vi "Configure Target - Legacy.vi"() -> ()   [LabVIEW 2020, in "LMH-LINX.lvlib"]
uses:
  LMH-LINX.lvlib
  Toolbox/LMH-Toolbox.lvlib
  Install LV Events.ctl
  Target Management/Install LV Data.ctl
  Target Management/Target Info.ctl
  Target Management/Status FGV States.ctl
  c:/p4/penguin/lvaddon/MakerHub/LINX/trunk/20.1/objects/MakerHub_LINX/win32U/i386/msvc90/release/LabVIEW/vi.lib/MakerHub/LINX/Resources/Renci.SshNet.dll
  Resources/Renci.SshNet.dll
  Target Management/NIC Info.ctl
  Target Management/NIC Mode.ctl
panel:
  in  "Done":bool
  out "Hostname":string
  out "Status":string
  in  "Hostname":string="raspberrypi"
  in  "Update Hostname":bool
  in  "Password":string="raspberry"
  in  "Username":string="pi"
  in  "Hostname or IP":string="raspberrypi"
  in  "Connect":bool
  out "Event Handler Iterations":i32
  out "Detailed Log":string
  out "Status Log":string
  out "Error Out":errorcluster
  # "Use this wizard to configure target settings for BeagleBone Black and Raspberry Pi 2 devices.\n\n1. Ensure the target is powered on and accessible on the same network as this computer.\n2. Enter the target's current hostname or IP address.\n3. Enter the new target hostname and click Update."
  # "Target Connection Settings"
  # "New Settings"
  # "LINX\nConfigure Target"
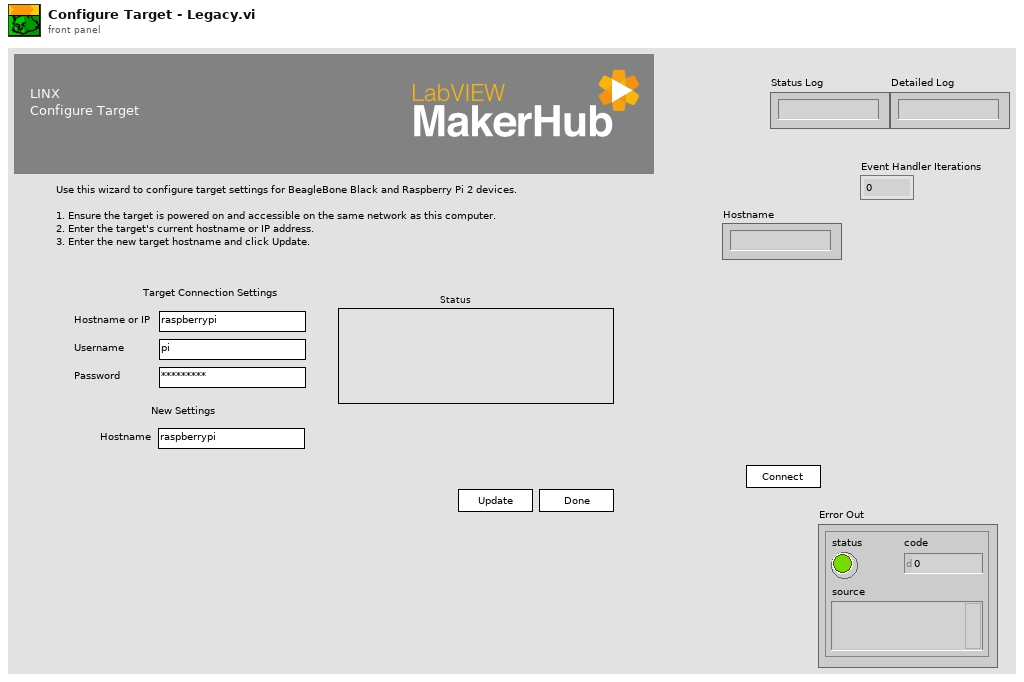
[diagram p1: front panel]
types:
  T1 = typedef "LMH-LINX.lvlib/Install LV Data.ctl" = cluster{"SSH Session":refnum<k24>, "Status Log":string, "Detailed Log":string, "Credentials":cluster{"Hostname or IP":string, "Username":string, "Password":string}, "Target Info":T2, "Reboot Required?":bool}
  T2 = typedef "LMH-LINX.lvlib/Target Info.ctl" = cluster{"OS Version":string, "CPU":string, "Systemd Version":string, "Internet Access":bool, "Device Type":string, "LV Installed Ver":string, "LV Available Ver":string, "LV Upgrade Available":bool, "Hostname":string, "NIC Info":T3[]}
  T3 = typedef "LMH-LINX.lvlib/NIC Info.ctl" = cluster{"Name":string, "NIC Mode":T4, "Configured":bool, "Config IP address":string, "Config Subnet mask":string, "Config Network":string, "Config gateway":string, "Wifi":bool, "SSID":string, "Password":string, "Configuration":string, "Current IP address":string, "Current Subnet mask":string, "Current gateway":string, "Current Network":string}
  T4 = typedef "LMH-LINX.lvlib/NIC Mode.ctl" = enum16{"DHCP", "Static", "Loopback"}
  T5 = typedef "LMH-LINX.lvlib/Install LV Events.ctl" = enum16{"Idle", "Connect", "Interrogate Device", "Pre Install", "Add MakerHub Feed", "Update Package Index", "Install LV", "Start LV", "Launch Example", "View Log", "Exit", "Update Hostname", "Menu: Target", "Menu: Install Software", "Menu: Network Settings", "Menu: Target Info", "NIC Select Change", "Menu: Network Settings Save", "Menu: Network Settings Cancel", "Menu: Cancel All"}
  T6 = typedef "LMH-LINX.lvlib/Status FGV States.ctl" = enum16{"Init", "Append", "Append History Only", "Set", "Get"}
  T7 = typedef "LMH-LINX.lvlib/Install LV Data.ctl" = cluster{"SSH Session":refnum<k1>, "Status Log":string, "Detailed Log":string, "Credentials":cluster{"Hostname or IP":string, "Username":string, "Password":string}, "Target Info":T2, "Reboot Required?":bool}
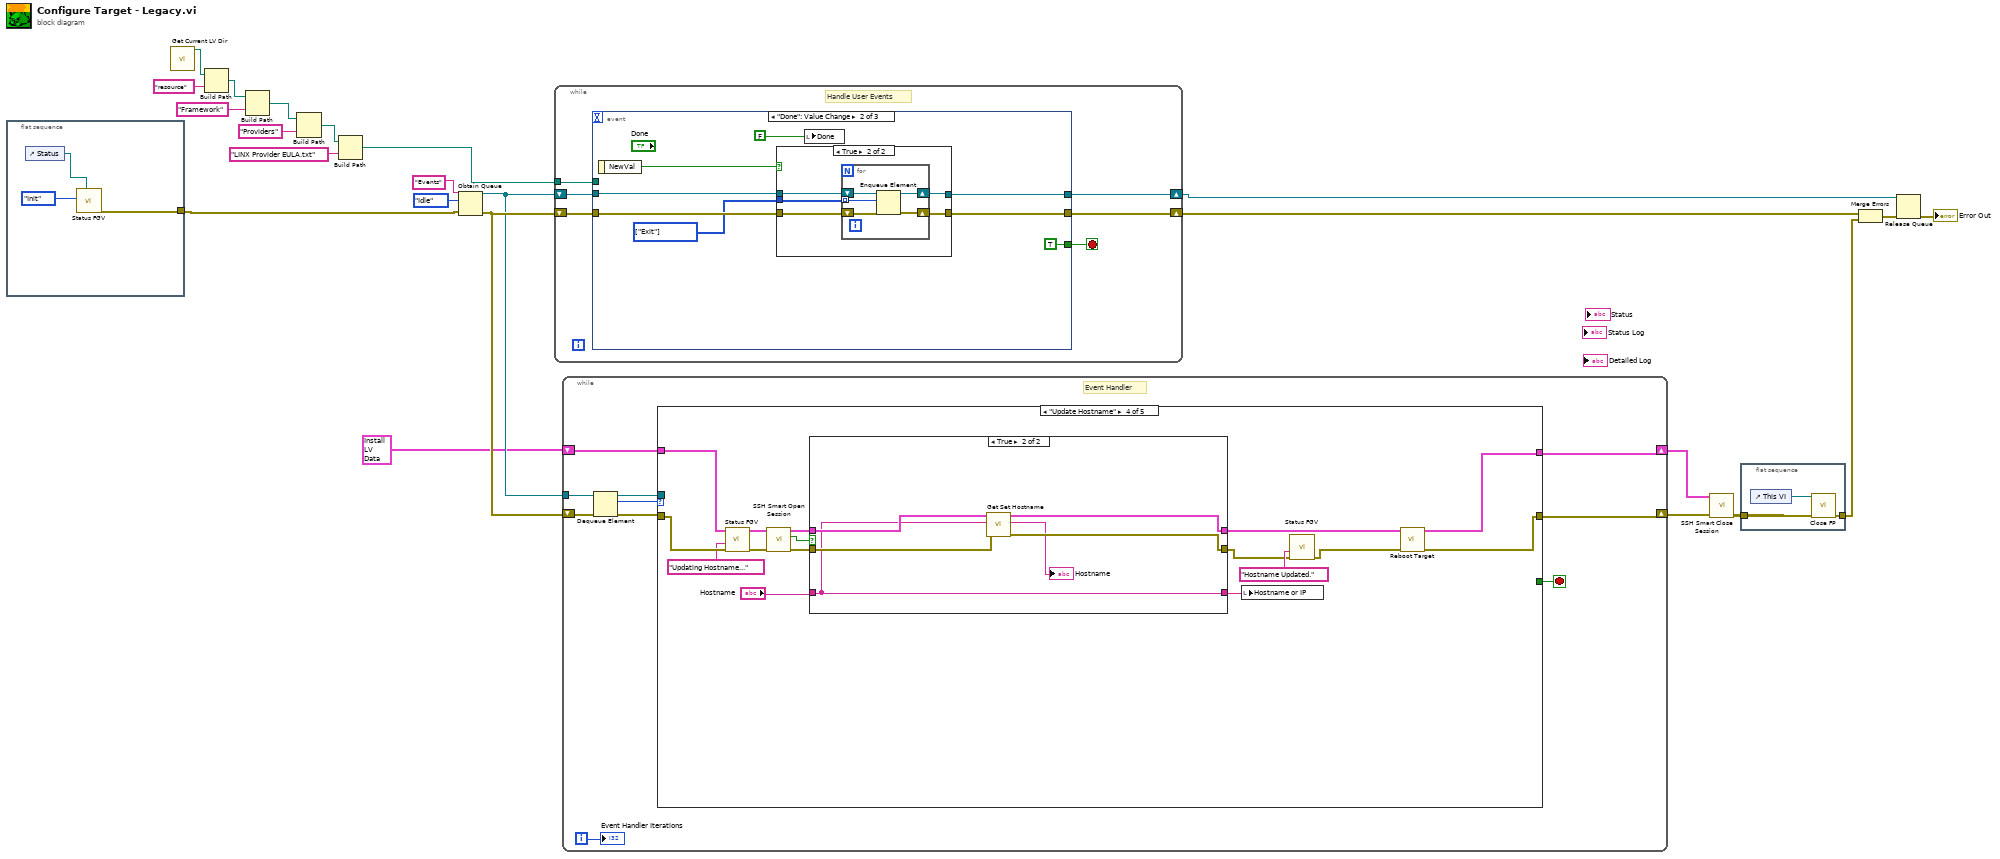
[diagram p0: block diagram]
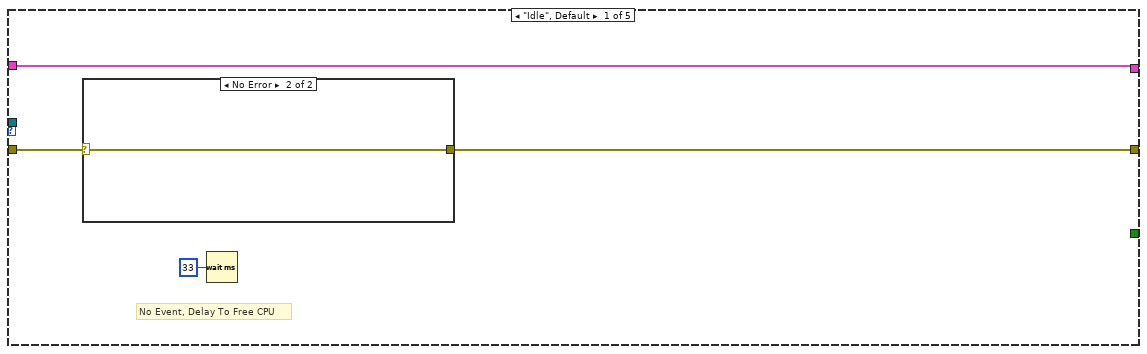
[diagram p2: hidden frame]
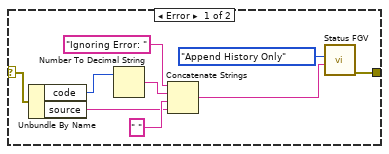
[diagram p3: hidden frame]
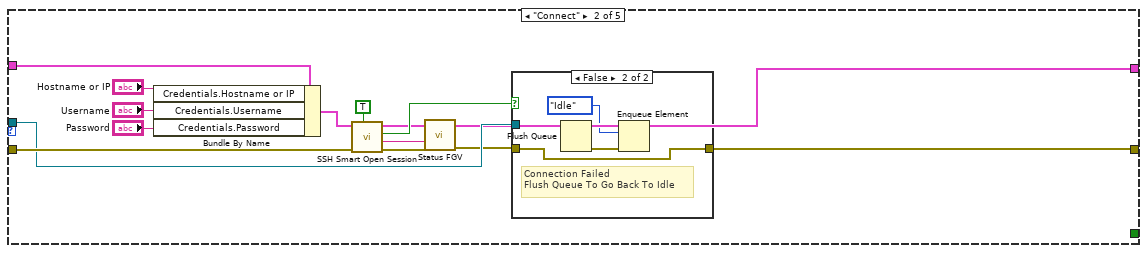
[diagram p4: hidden frame]
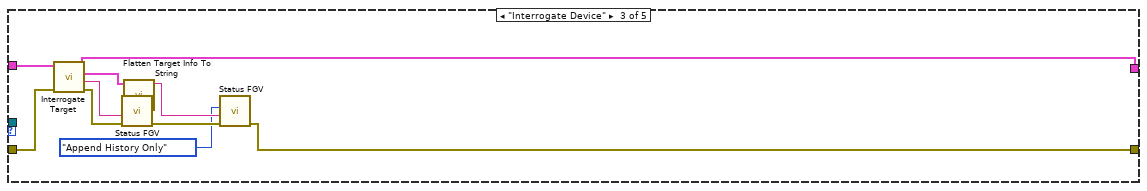
[diagram p6: hidden frame]
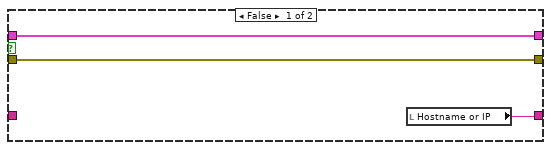
[diagram p7: hidden frame]
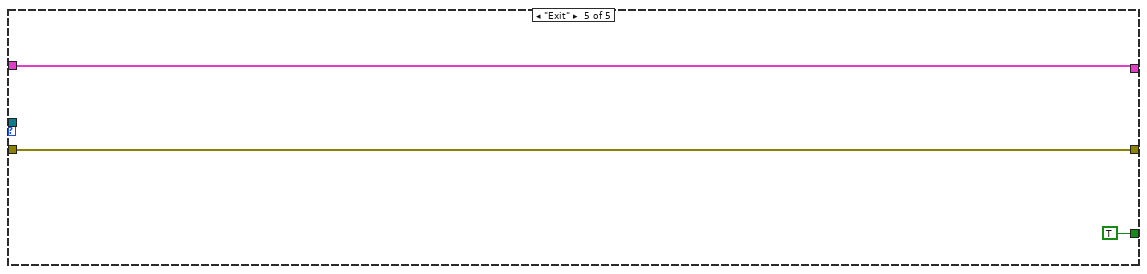
[diagram p8: hidden frame]
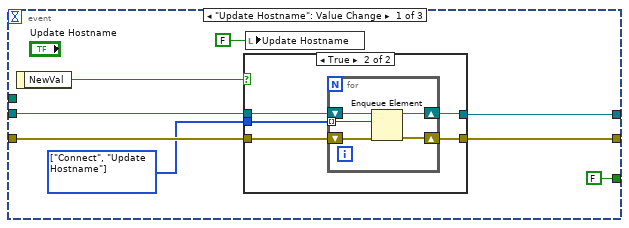
[diagram p9: hidden frame]
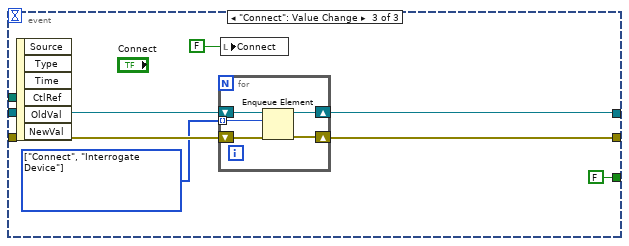
[diagram p12: hidden frame]
diagram:
  n1 = flat-sequence {
    tunnel: [w25] -> w1
    frame #0 {
      n2 = control-ref of="Status"() -> (w24:refnum<vi>)
      n3 = call "Status FGV.vi"("Live Status Ref"=w24, "Status FGV State"=Status_FGV_States."Init") -> ("Error Out"=w25:errorcluster)  [unwired: 7 in, 2 out]
    }
  }
  n4 = call "Get Current LV Dir.vi"() -> ("This LV Directory"=w23:path)  [unwired: 10 in, 1 out]
  n5 = Build Path(base path=w23, name or relative path="resource") -> (appended path=w16:path)
  n6 = Build Path(base path=w16, name or relative path="Framework") -> (appended path=w17:path)
  n7 = Build Path(base path=w17, name or relative path="Providers") -> (appended path=w18:path)
  n8 = Build Path(base path=w18, name or relative path="LINX Provider EULA.txt") -> (appended path=w15:path)
  n9 = Obtain Queue(name (unnamed)="Events", element data type=Install_LV_Events."Idle" ("Install LV Support State"), error in (no error)=w1) -> (queue out=w12:refnum<queue>, error out=w13:errorcluster)  [unwired: 2 in, 1 out]
  n10 = while {
    shift-right: [w31] -> w3
    shift-left: w13 -> [w32]
    tunnel: w15 -> [w29]
    shift-right: [w28] -> w8
    shift-left: w12 -> [w27]
    stop <- w30 stop-if-true
    # "Handle User Events"
    n11 = event shown="[1] \"Done\": Value Change" {
      selector: _ -> [_ _ _]
      dyn-events: _ -> [_ _ _]
      timeout: _ -> [_ _ _]
      tunnel: [w37 w57 w75] -> w31
      tunnel: w32 -> [w38 w58 w74]
      tunnel: [FALSE TRUE FALSE] -> w30
      tunnel: w29 -> [_ _ _]
      tunnel: [w36 w56 w76] -> w28
      tunnel: w27 -> [w35 w55 w77]
      event "Update Hostname": Value Change {
        w34 = T5[] [enum."Connect", enum."Update Hostname"] items=["Idle", "Connect", "Interrogate Device", "Pre Install", "Add MakerHub Feed", "Update Package Index", "Install LV", "Start LV", "Launch Example", "View Log", "Exit", "Update Hostname", "Menu: Target", "Menu: Install Software", "Menu: Network Settings", "Menu: Target Info", "NIC Select Change", "Menu: Network Settings Save", "Menu: Network Settings Cancel", "Menu: Cancel All"]
        n12 = event-data() -> ("NewVal"=w33:bool)  [unwired: 1 in]
        n13 = case shown="True" w33 {
          tunnel: w38 -> [w42 w47]
          tunnel: [w42 w46] -> w37
          tunnel: [w41 w45] -> w36
          tunnel: w35 -> [w41 w44]
          tunnel: w34 -> [_ w43]
          frame False {
            # "Ignore Change \nto False"
          }
          frame True {
            n14 = for {
              shift-right: [w51] -> w46
              shift-left: w47 -> [w52]
              shift-right: [w50] -> w45
              shift-left: w44 -> [w49]
              tunnel: w43 -> [w48] mode=indexing
              n15 = Enqueue Element(queue=w49, element=w48, error in (no error)=w52) -> (queue out=w50:refnum<queue>, error out=w51:errorcluster)  [unwired: 1 in, 1 out]
            }
          }
        }
        n16 = local write "Update Hostname"(FALSE ("Install")) -> ()
      }
      event "Done": Value Change {
        w54 = T5[] [enum."Exit"] items=["Idle", "Connect", "Interrogate Device", "Pre Install", "Add MakerHub Feed", "Update Package Index", "Install LV", "Start LV", "Launch Example", "View Log", "Exit", "Update Hostname", "Menu: Target", "Menu: Install Software", "Menu: Network Settings", "Menu: Target Info", "NIC Select Change", "Menu: Network Settings Save", "Menu: Network Settings Cancel", "Menu: Cancel All"]
        n17 = event-data() -> ("NewVal"=w53:bool)  [unwired: 1 in]
        n18 = case shown="True" w53 {
          tunnel: w58 -> [w62 w67]
          tunnel: [w62 w66] -> w57
          tunnel: [w61 w65] -> w56
          tunnel: w55 -> [w61 w64]
          tunnel: w54 -> [_ w63]
          frame False {
            # "Ignore Change \nto False"
          }
          frame True {
            n19 = for {
              shift-right: [w71] -> w66
              shift-left: w67 -> [w72]
              shift-right: [w70] -> w65
              shift-left: w64 -> [w69]
              tunnel: w63 -> [w68] mode=indexing
              n20 = Enqueue Element(queue=w69, element=w68, error in (no error)=w72) -> (queue out=w70:refnum<queue>, error out=w71:errorcluster)  [unwired: 1 in, 1 out]
            }
          }
        }
        n21 = local write "Done"(FALSE ("Install")) -> ()
      }
      event "Connect": Value Change {
        w73 = T5[] [enum."Connect", enum."Interrogate Device"] items=["Idle", "Connect", "Interrogate Device", "Pre Install", "Add MakerHub Feed", "Update Package Index", "Install LV", "Start LV", "Launch Example", "View Log", "Exit", "Update Hostname", "Menu: Target", "Menu: Install Software", "Menu: Network Settings", "Menu: Target Info", "NIC Select Change", "Menu: Network Settings Save", "Menu: Network Settings Cancel", "Menu: Cancel All"]
        n22 = event-data() -> ()  [unwired: 1 in, 6 out]
        n23 = for {
          shift-right: [w83] -> w75
          shift-left: w74 -> [w84]
          shift-right: [w82] -> w76
          shift-left: w77 -> [w81]
          tunnel: w73 -> [w80] mode=indexing
          n24 = Enqueue Element(queue=w81, element=w80, error in (no error)=w84) -> (queue out=w82:refnum<queue>, error out=w83:errorcluster)  [unwired: 1 in, 1 out]
        }
        n25 = local write "Connect"(FALSE ("Interrogate")) -> ()
      }
    }
  }
  n26 = while {
    shift-right: [w93] -> w7
    shift-left: w13 -> [w91]
    tunnel: w12 -> [w92]
    shift-right: [w88] -> w2
    shift-left: T1 {"SSH Session"=refnum, "Status Log"="", "Detailed Log"="", "Credentials"={"Hostname or IP"="", "Username"="", "Password"=""}, "Target Info"={"OS Version"="", "CPU"="", "Systemd Version"="", "Internet Access"=FALSE, "Device Type"="", "LV Installed Ver"="", "LV Available Ver"="", "LV Upgrade Available"=FALSE, "Hostname"="", "NIC Info"=[]}, "Reboot Required?"=FALSE} ("Install LV Data") -> [w86]
    i -> [w87]
    stop <- w94 stop-if-true
    # "Event Handler"
    n27 = Dequeue Element(queue=w92, error in (no error)=w91) -> (queue out=w85:refnum<queue>, element=w89:T5, error out=w90:errorcluster)  [unwired: 1 in, 1 out]
    n28 = case shown="\"Update Hostname\"" w89 {
      tunnel: [w95 w118 w129 w148 w164] -> w93
      tunnel: w90 -> [w96 w122 w138 w146 w164]
      tunnel: [_ _ _ _ TRUE] -> w94
      tunnel: [w97 w109 w130 w147 w163] -> w88
      tunnel: w86 -> [w97 w111 w131 w153 w163]
      tunnel: w85 -> [_ w119 _ _ _]
      frame "Idle", Default {
        # "No Event, Delay To Free CPU"
        n29 = case shown="No Error" w96 {
          selector: w96 -> [w106 w108]
          tunnel: [w107 w108] -> w95
          frame Error {
            n30 = Unbundle By Name(w106) -> ("code"=w104:i32, "source"=w101:string)
            n31 = Number To Decimal String(number=w104) -> (decimal integer string=w103:string)  [unwired: 1 in]
            n32 = Concatenate Strings("Ignoring Error: " ("Status"), w103, " " ("string"), w101) -> (w100:string)
            n33 = call "Status FGV.vi"("Status"=w100, "Status FGV State"=Status_FGV_States."Append History Only") -> ("Error Out"=w107:errorcluster)  [unwired: 7 in, 2 out]
          }
          frame No Error {
          }
        }
        n34 = Wait (ms)(milliseconds to wait=u32 33) -> ()  [unwired: 1 out]
      }
      frame "Connect" {
        n35 = Bundle By Name(cluster=w111, "Credentials.Hostname or IP"="Hostname or IP", "Credentials.Username"="Username", "Credentials.Password"="Password") -> (w110:T1)
        n36 = call "SSH Smart Open Session.vi"("Force Reconnect?"=TRUE, "Error In"=w122, "Install LV Data in"=w110) -> ("Error Out"=w117:errorcluster, "Status"=w115:string, "Connected?"=w120:bool, "Install LV Data out"=w109:T7)  [unwired: 5 in]
        n37 = call "Status FGV.vi"("Error In"=w117, "Status"=w115) -> ("Error Out"=w116:errorcluster)  [unwired: 7 in, 2 out]
        n38 = case shown="False" w120 {
          tunnel: w119 -> [_ w128]
          tunnel: w116 -> [w123 w124]
          tunnel: [w123 w124] -> w118
          frame True {
          }
          frame False {
            # "Connection Failed\nFlush Queue To Go Back To Idle"
            n39 = Flush Queue(queue=w128) -> (queue out=w126:refnum<queue>, error out=w127:errorcluster)  [unwired: 1 in, 1 out]
            n40 = Enqueue Element(queue=w126, element=Install_LV_Events."Idle", error in (no error)=w127) -> ()  [unwired: 1 in, 3 out]
          }
        }
      }
      frame "Interrogate Device" {
        n41 = call "Interrogate Target.vi"("Error In"=w138, "Install LV Data"=w131) -> ("Error Out"=w137:errorcluster, "Status"=w136:string, "Target Info"=w135:T2, "Install LV Data"=w130:T7)  [unwired: 6 in]
        n42 = call "Status FGV.vi"("Error In"=w137, "Status"=w136) -> ("Error Out"=w133:errorcluster)  [unwired: 7 in, 2 out]
        n43 = call "Flatten Target Info To String.vi"("Target Info"=w135) -> ("Target Info String"=w134:string)  [unwired: 10 in]
        n44 = call "Status FGV.vi"("Error In"=w133, "Status"=w134, "Status FGV State"=Status_FGV_States."Append History Only") -> ("Error Out"=w129:errorcluster)  [unwired: 6 in, 2 out]
      }
      frame "Update Hostname" {
        n45 = call "Status FGV.vi"("Error In"=w146, "Status"="Updating Hostname...") -> ("Error Out"=w145:errorcluster)  [unwired: 7 in, 2 out]
        n46 = call "SSH Smart Open Session.vi"("Error In"=w145, "Install LV Data in"=w153) -> ("Error Out"=w151:errorcluster, "Connected?"=w152:bool, "Install LV Data out"=w150:T7)  [unwired: 6 in, 1 out]
        n47 = case shown="True" w152 {
          tunnel: w151 -> [w155 w162]
          tunnel: w150 -> [w156 w161]
          tunnel: [w155 w160] -> w142
          tunnel: [w156 w159] -> w141
          tunnel: "Hostname" -> [_ w158]
          tunnel: [w154 w158] -> w139
          frame False {
            n48 = local read "Hostname or IP"() -> (w154:string)
          }
          frame True {
            n49 = call "Get Set Hostname.vi"("Error In"=w162, "Hostname"=w158, "Install LV Data"=w161) -> ("Error Out"=w160:errorcluster, "Hostname"=→"Hostname":string, "Install LV Data"=w159:T7)  [unwired: 6 in]
          }
        }
        n50 = local write "Hostname or IP"(w139) -> ()
        n51 = call "Status FGV.vi"("Error In"=w142, "Status"="Hostname Updated.") -> ("Error Out"=w140:errorcluster)  [unwired: 7 in, 2 out]
        n52 = call "Reboot Target.vi"("Error In"=w140, "Install LV Data"=w141) -> ("Error Out"=w148:errorcluster, "Install LV Data"=w147:T7)  [unwired: 7 in, 1 out]
      }
      frame "Exit" {
      }
    }
    "Event Handler Iterations" <- w87
  }
  n53 = call "SSH Smart Close Session.vi"("Error In"=w7, "Install LV Data"=w2) -> ("Error Out"=w4:errorcluster)  [unwired: 8 in, 1 out]
  n54 = flat-sequence {
    tunnel: [w167] -> w6
    tunnel: w4 -> [w166]
    frame #0 {
      n55 = control-ref of="This VI"() -> (w168:refnum<vi>)
      n56 = call "Close FP.vi"("Error In"=w166, "VI Ref"=w168) -> ("Error Out"=w167:errorcluster)  [unwired: 9 in]
    }
  }
  n57 = Merge Errors(w3, w6) -> (w9:errorcluster)
  n58 = Release Queue(queue=w8, error in (no error)=w9) -> (error out=→"Error Out":errorcluster)  [unwired: 1 in, 2 out]
